vi "Print.vi"(8 "error in (no error)":errorcluster caption="entrée d'erreur (pas d'erreur)", 11 "Class Printer (Default) en entrée":refnum<class "Class Printer (Default).lvclass">) -> (0 "error out":errorcluster caption="sortie d'erreur", 3 "Class Printer (Default) en sortie":refnum<class "Class Printer (Default).lvclass">)   [LabVIEW 2020, in "Library Instrument & Equipement.lvlib" / "Library Printer.lvlib" / "Class Printer (Default).lvclass"]
uses:
  Class Printer (Default).lvclass
  Commun VI/TypeDef/Variable Printable.ctl
  Class Printer (Default).lvclass/Class Printer (Default).ctl
  Commun VI/Library Commun.lvlib
panel:
  in  "Variable":T1="$Batch$"
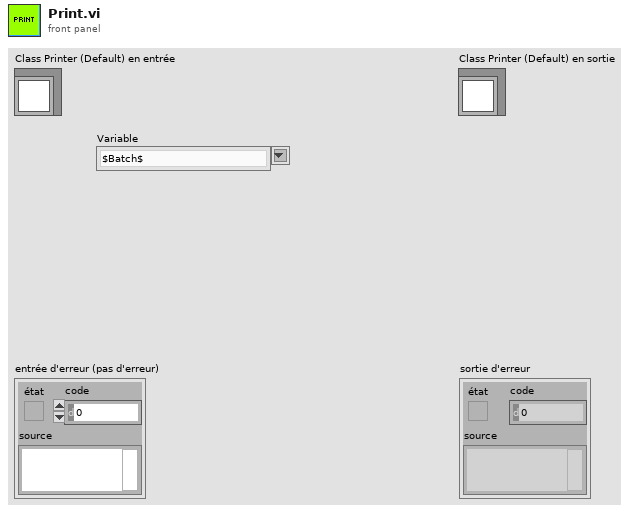
[diagram p1: front panel]
types:
  T1 = typedef "Variable Printable.ctl" = string
  T2 = enum16{"Get Variable", "Get All Variables", "Set Variable", "Delete Variable", "Delete All Variable"}
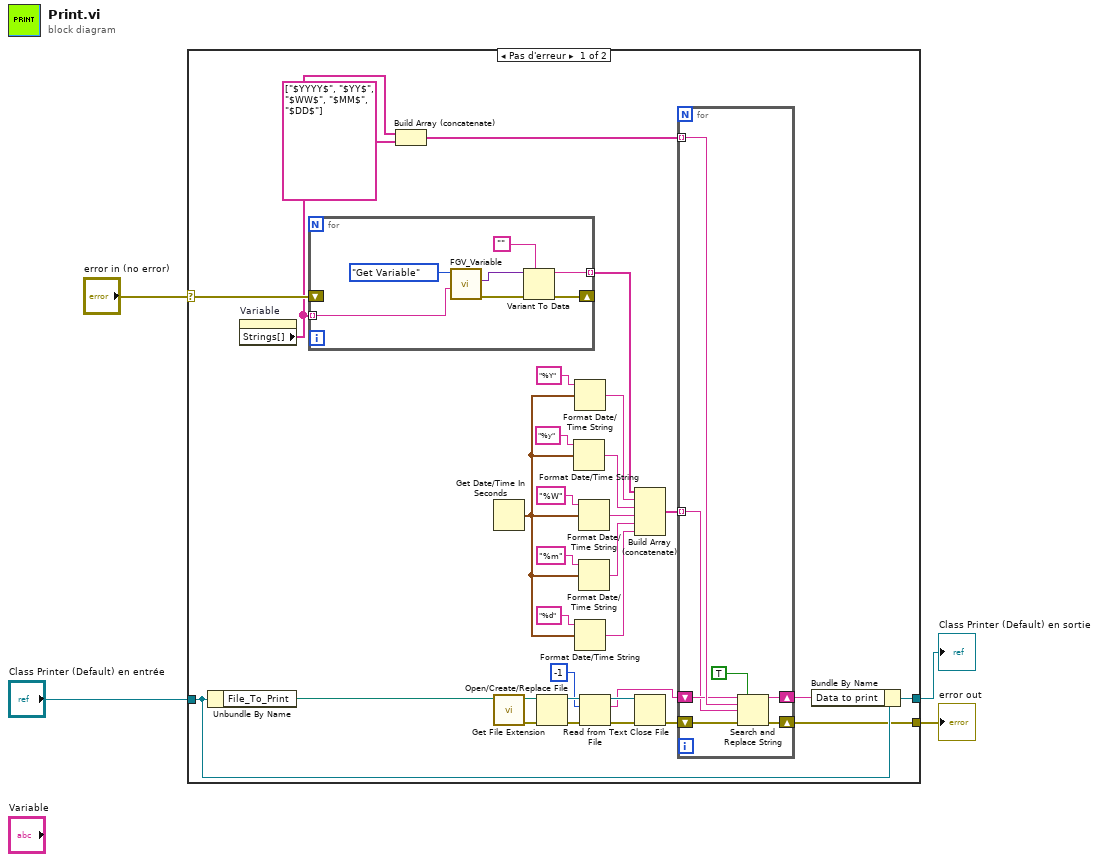
[diagram p0: block diagram]
diagram:
  n1 = case shown="Pas d'erreur" "error in (no error)" {
    selector: "error in (no error)" -> [w16 w51]
    tunnel: [w17 w51] -> w3
    tunnel: [w26 w50] -> w1
    tunnel: "Class Printer (Default) en entrée" -> [w27 w50]
    frame No Error {
      n2 = Unbundle By Name(w27) -> ("File_To_Print"=w28:path)
      n3 = property on="Variable" class="ChneDér (strict)"() -> ("Strings[]"=w14:string[])  [unwired: 2 in, 2 out]
      n4 = for {
        tunnel: w14 -> [w36] mode=indexing
        shift-right: [w40] -> _
        shift-left: w16 -> [_]
        tunnel: [w37] -> w13 mode=indexing
        n5 = call "FGV_Variable.vi"("Variable"=w36, "Function"=T2."Get Variable") -> ("error out"=w41:errorcluster, "Data Out"=w39:variant)  [unwired: 7 in, 1 out]
        n6 = Variant To Data(error in=w41, type="", Variant=w39) -> (data=w37:string, error out=w40:errorcluster)
      }
      n7 = Build Array (concatenate)(w14, string[] ["$YYYY$", "$YY$", "$WW$", "$MM$", "$DD$"]) -> (w12:string[])
      n8 = Get Date/Time In Seconds() -> (seconds since 1Jan1904=w7:timestamp)
      n9 = call <vilib>:"Get File Extension.vi"("file"=w28) -> ("error out"=w29:errorcluster, "dup file"=w30:path)  [unwired: 6 in, 3 out]
      n10 = Open/Create/Replace File(file path (use dialog)=w30, error in=w29) -> (refnum out=w35:refnum<file>, error out=w33:errorcluster)  [unwired: 4 in, 1 out]
      n11 = Format Date/Time String(time format string (%c)="%y" ("chaîne de format de l'heure (%c)"), seconds (now)=w7) -> (date/time string=w22:string)  [unwired: 1 in]
      n12 = Format Date/Time String(time format string (%c)="%Y" ("chaîne de format de l'heure (%c)"), seconds (now)=w7) -> (date/time string=w5:string)  [unwired: 1 in]
      n13 = Format Date/Time String(time format string (%c)="%d" ("chaîne de format de l'heure (%c)"), seconds (now)=w7) -> (date/time string=w8:string)  [unwired: 1 in]
      n14 = Format Date/Time String(time format string (%c)="%W" ("chaîne de format de l'heure (%c)"), seconds (now)=w7) -> (date/time string=w21:string)  [unwired: 1 in]
      n15 = Format Date/Time String(time format string (%c)="%m" ("chaîne de format de l'heure (%c)"), seconds (now)=w7) -> (date/time string=w11:string)  [unwired: 1 in]
      n16 = Read from Text File(file (use dialog)=w35, count=-1 ("nombre"), error in=w33) -> (refnum out=w31:refnum<file>, text=w20:string, error out=w32:errorcluster)  [unwired: 1 in, 1 out]
      n17 = Build Array (concatenate)(w13, w5, w22, w21, w11, w8) -> (w23:string[])
      n18 = Close File(refnum=w31, error in=w32) -> (error out=w18:errorcluster)  [unwired: 1 out]
      n19 = for {
        tunnel: w12 -> [w49] mode=indexing
        shift-right: [w46] -> w17
        shift-left: w18 -> [w48]
        shift-right: [w45] -> w19
        shift-left: w20 -> [w47]
        tunnel: w23 -> [w43] mode=indexing
        n20 = Search and Replace String(replace all?=TRUE ("tout remplacer ? (F)"), input string=w47, search string=w49, replace string=w43, error in=w48) -> (result string=w45:string, error out=w46:errorcluster)  [unwired: 3 in, 2 out]
      }
      n21 = Bundle By Name(cluster=w27, "Data to print"=w19) -> (w26:refnum<class "Class Printer (Default).lvclass">)
    }
    frame Error {
    }
  }
  "error out" <- w3
  "Class Printer (Default) en sortie" <- w1
